vi "frame_sel_v2.vi"(8 "正则表达式":string, 10 "帧长":i32, 11 "输入字符串":string) -> ()   [LabVIEW 2012]
panel:
  out "输入字符串 3":string
  out "输入字符串 2":string
  out "数值":i32
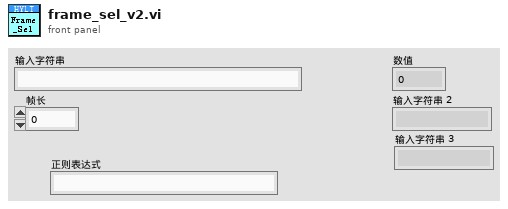
[diagram p1: front panel]
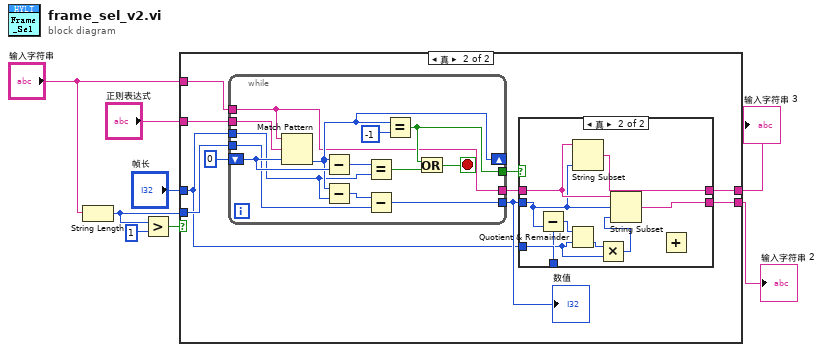
[diagram p0: block diagram]
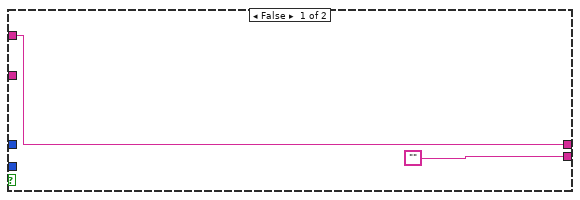
[diagram p2: hidden frame]
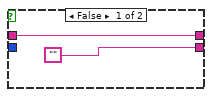
[diagram p3: hidden frame]
diagram:
  n1 = String Length(string="输入字符串") -> (length=w3:i32)
  n2 = Greater?(x=w3, y=1) -> (0:w4:bool)
  n3 = case shown="真" w4 {
    tunnel: "正则表达式" -> [_ w19]
    tunnel: "帧长" -> [_ w11]
    tunnel: "输入字符串" -> [w10 w20]
    tunnel: w3 -> [_ w15]
    tunnel: ["" w13] -> w2
    tunnel: [w10 w12] -> w1
    frame False {
    }
    frame True {
      n4 = while {
        tunnel: [w32] -> w17
        tunnel: w20 -> [w32]
        tunnel: w19 -> [w36]
        shift-right: [w40] -> _
        shift-left: 0 ("offset past match") -> [w42]
        tunnel: w11 -> [w39]
        tunnel: [w38] -> w16
        tunnel: w15 -> [w34]
        tunnel: [w33] -> w14
        stop <- w43 stop-if-true
        n5 = Match Pattern(string=w32, regular expression=w36, offset (0)=w42) -> (offset past match=w40:i32)  [unwired: 3 out]
        n6 = Subtract(x=w40, y=w42) -> (x-y=w41:i32)
        n7 = Subtract(x=w40, y=w39) -> (x-y=w37:i32)
        n8 = Equal?(x=w41, y=w39) -> (x = y?=w35:bool)
        n9 = Subtract(x=w37, y=w34) -> (x-y=w38:i32)
        n10 = Equal?(x=w40, y=-1) -> (x = y?=w33:bool)
        n11 = Or(x=w33, y=w35) -> (x .or. y?=w43:bool)
      }
      "数值" <- w16
      n12 = case shown="真" w14 {
        tunnel: w17 -> [w22 w30]
        tunnel: w16 -> [_ w27]
        tunnel: ["" w31] -> w13
        tunnel: [w22 w29] -> w12
        tunnel: w11 -> [_ w28]
        tunnel: w11 -> [_ w24]
        frame False {
        }
        frame True {
          n13 = Subtract(x=w28, y=w27) -> (x-y=w26:i32)
          n14 = Quotient & Remainder(x=w26, y=w24) -> (floor(x/y)=w25:i32)  [unwired: 1 out]
          n15 = String Subset(string=w30, length (rest)=w27) -> (substring=w29:string)  [unwired: 1 in]
          n16 = Multiply(x=w25, y=w24) -> (x*y=w23:i32)
          n17 = String Subset(string=w30, offset (0)=w27, length (rest)=w23) -> (substring=w31:string)
          n18 = Add() -> ()  [unwired: 2 in, 1 out]
        }
      }
    }
  }
  "输入字符串 2" <- w2
  "输入字符串 3" <- w1
